vi "Upright_Start.vi"(10 "IMU_sample_rate":i32=200, 11 "Current Theta":dbl) -> (3 "Upright Counter":dbl)   [LabVIEW 2014]
uses:
  Start.vi
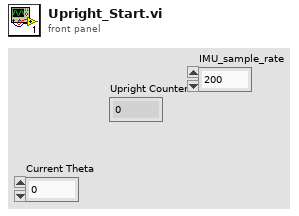
[diagram p1: front panel]
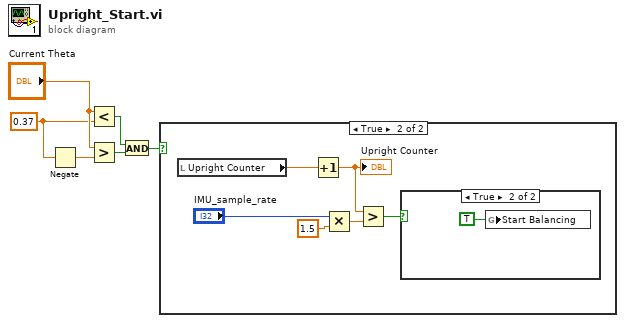
[diagram p0: block diagram]
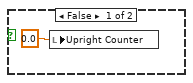
[diagram p2: hidden frame]
diagram:
  w4 = 0.37
  n1 = Negate(x=w4) -> (-x=w3:dbl)
  n2 = Less?(x="Current Theta", y=w4) -> (x < y?=w2:bool)
  n3 = Greater?(x="Current Theta", y=w3) -> (0:w1:bool)
  n4 = And(x=w2, y=w1) -> (x .and. y?=w6:bool)
  n5 = case shown="True" w6 {
    frame False {
      n6 = local write "Upright Counter"(0.0 ("Upright Counter")) -> ()
    }
    frame True {
      n7 = local read "Upright Counter"() -> (w11:dbl)
      n8 = Increment(x=w11) -> (x+1=w12:dbl)
      "Upright Counter" <- w12
      n9 = Multiply(x="IMU_sample_rate", y=1.5) -> (x*y=w8:dbl)
      n10 = Greater?(x=w12, y=w8) -> (0:w13:bool)
      n11 = case shown="True" w13 {
        frame False {
        }
        frame True {
          n12 = global write "Start.vi" "Start Balancing"(TRUE) -> ()
        }
      }
    }
  }
